vi "GyroForwardUltrasonic.vi"(11 "Ultrasonic Distance":dbl) -> ()   [LabVIEW 2016, in "LEGO-PMR.lvrbt"]
uses:
  LEGO-PMR.lvrbt
  <vilib>/NXT/Block Support/NXT_InputPort.ctl
  <vilib>/NXT/Block Support/NXT_OutputPort.ctl
  <vilib>/NXT/LegoClasses/BrickReference/BrickReference.lvclass
  <vilib>/NXT/Subs/LVHSConnector.ctl
  <vilib>/NXT/NXTIO Xnodes/NXTIONodeSubVIs/NXTMoveMotors.vi
  <vilib>/NXT/NXTIO Xnodes/NXTIOXNode/NXTIO.xnode
  <vilib>/NXT/NXTIO Xnodes/AddressXNode/NXTIOAddress.xnode
  <vilib>/NXT/Dual Mode Library/Waits/Wait_Num(msec).vi
  <vilib>/NXT/Dual Mode Library/Sensors/EV3_Gyro_Angle.vi
  <vilib>/NXT/Dual Mode Library/Sensors/EV3_Ultrasonic_CM.vi
panel:
  out "Read Angle 2":dbl
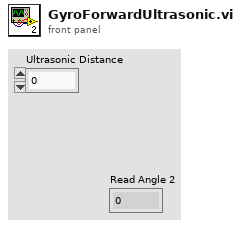
[diagram p1: front panel]
types:
  T1 = typedef "NXT_OutputPort.ctl" = u8
  T2 = typedef "NXT_InputPort.ctl" = u32
  T3 = typedef "LVHSConnector.ctl" = refnum<class "BrickReference.lvclass">
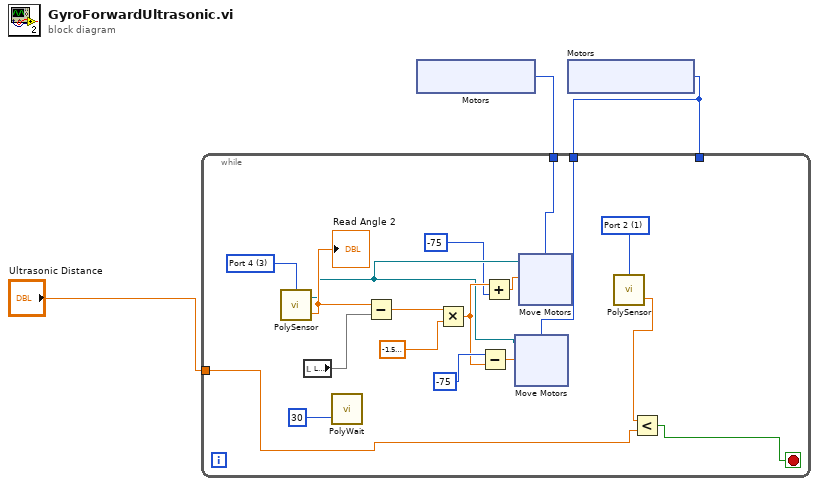
[diagram p0: block diagram]
diagram:
  n1 = xnode "Motors"() -> ("Motor"=w3:T1)
  n2 = xnode "Motors"() -> ("Motor"=w2:T1)
  n3 = while {
    tunnel: w3 -> [w16]
    tunnel: w2 -> [w15]
    tunnel: w2 -> [_]
    tunnel: "Ultrasonic Distance" -> [w4]
    stop <- w6 stop-if-true
    w7 = T2 1 items=["Port 1", "Port 2", "Port 3", "Port 4"] ("Port (Port 1)")
    w21 = T2 3 items=["Port 1", "Port 2", "Port 3", "Port 4"] ("Port (Port 1)")
    n4 = call-poly <vilib>:"PolySensor.vi"("Port (Port 1)"=w21) -> ("Degrees"=w17:sgl, "NXT/EV3"=w9:T3)  [unwired: 2 in]
    "Read Angle 2" <- w17
    n5 = local read item#-1() -> (w20)
    n6 = call-poly <vilib>:"PolyWait.vi"("Time (100 msec)"=u32 30 ("Time (1 sec)")) -> ()  [unwired: 3 in, 1 out]
    n7 = Subtract(x=w17, y=w20) -> (x-y=w18:sgl)
    n8 = Multiply(x=w18, y=-1.5000000000000002) -> (x*y=w12:dbl)
    n9 = Subtract(x=-75, y=w12) -> (x-y=w11:dbl)
    n10 = Add(x=w12, y=-75) -> (x+y=w10:dbl)
    n11 = xnode "Move Motors"("Power/Speed 1"=w11, "Motors"=w15, "NXT/EV3"=w9) -> ()  [unwired: 1 out]
    n12 = xnode "Move Motors"("Power/Speed 1"=w10, "Motors"=w16, "NXT/EV3"=w9) -> ()  [unwired: 1 out]
    n13 = call-poly <vilib>:"PolySensor.vi"("Port (Port 1)"=w7) -> ("Centimeters"=w5:sgl)  [unwired: 2 in, 1 out]
    n14 = Less?(x=w5, y=w4) -> (x < y?=w6:bool)
  }
